vi "GetTagsForPreferences.vi"(3 "Default":u16, 4 "Tag":string, 5 "File":string) -> (0 "tag":string, 2 "tag value":i32)   [LabVIEW 2014]
doc: "Gets tag and returns tag value"
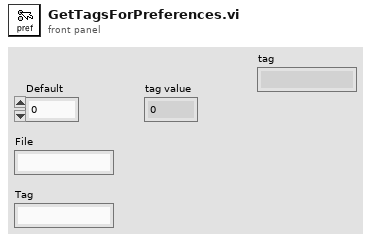
[diagram p1: front panel]
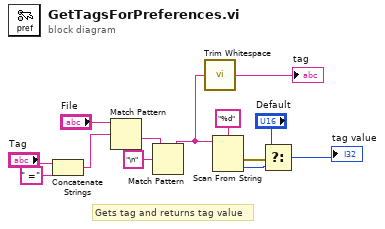
[diagram p0: block diagram]
diagram:
  # "Gets tag and returns tag value"
  n1 = Concatenate Strings("Tag", " =" ("string")) -> (w5:string)
  n2 = Match Pattern(string="File", regular expression=w5) -> (after substring=w4:string)  [unwired: 1 in, 3 out]
  n3 = Match Pattern(string=w4, regular expression="\n") -> (before substring=w2:string)  [unwired: 1 in, 3 out]
  n4 = call <vilib>:"Trim Whitespace.vi"("string"=w2) -> ("trimmed string"=→"tag":string)  [unwired: 1 in]
  n5 = Scan From String(format string="%d", input string=w2) -> (error out=w9:errorcluster, output 1=w10:i32)  [unwired: 3 in, 2 out]
  n6 = Select(t="Default", s=w9, f=w10) -> (s? t:f=→"tag value":i32)
